vi "GetPower.vi"(4 "error in (no error)":errorcluster, 5 "Measeaurement mode":string(combo)="PM100D", 6 "Wavelength (nm)":dbl=350.0 min=350.0 max=1100.0 format="%#.1f", 7 "Input Device":refnum<visa-resource-name>) -> (0 "error out":errorcluster, 1 "Power (W)":dbl, 2 "Responsivity (A/W)":dbl, 3 "VISA Resource Name out":refnum<visa-resource-name>="GPIB0::22::INSTR")   [LabVIEW 2011]
uses:
  <vilib>/Utility/file.llb/Read From Spreadsheet File (DBL).vi
panel:
  out "Det36A responsivity":dbl[](array[numeric])
  out "Wavelength":dbl[](array[numeric])
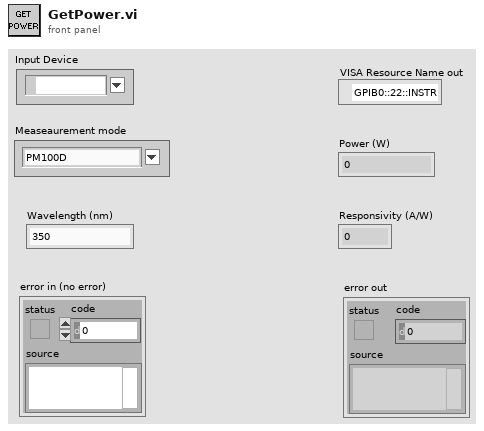
[diagram p1: front panel]
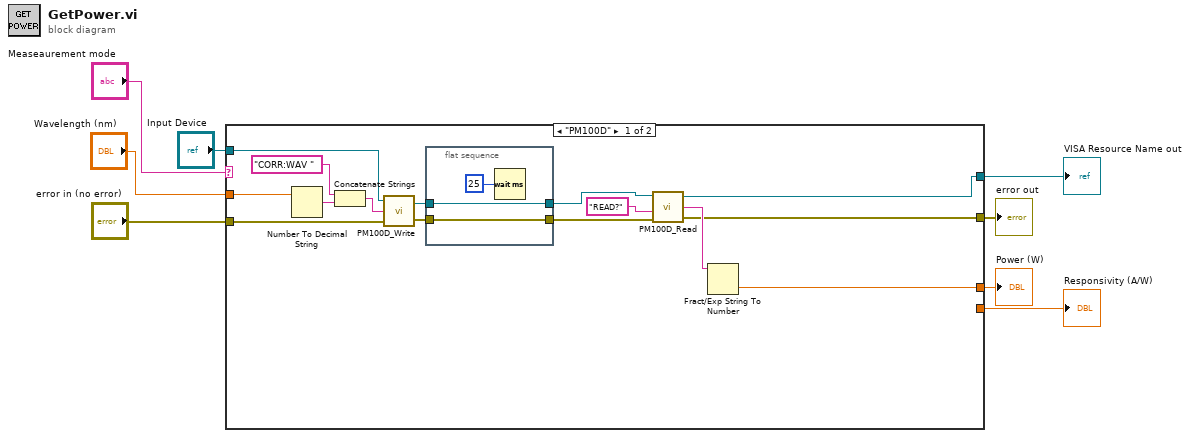
[diagram p0: block diagram]
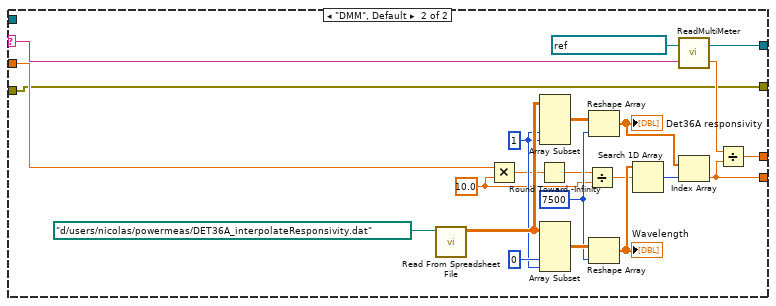
[diagram p2: hidden frame]
diagram:
  n1 = case shown="\"PM100D\"" "Measeaurement mode" {
    selector: "Measeaurement mode" -> [_ w29]
    tunnel: "Input Device" -> [w17 _]
    tunnel: [_ w37] -> w7
    tunnel: [w15 w36] -> w6
    tunnel: "Wavelength (nm)" -> [w19 w35]
    tunnel: [w21 w30] -> w4
    tunnel: [w12 w27] -> w2
    tunnel: "error in (no error)" -> [w9 w27]
    frame "PM100D" {
      n2 = Number To Decimal String(number=w19) -> (decimal integer string=w20:string)  [unwired: 1 in]
      n3 = Concatenate Strings("CORR:WAV " ("chaîne"), w20) -> (w16:string)
      n4 = call "PM100D_Write.vi"("error in (no error)"=w9, "Command"=w16, "VISA in"=w17) -> ("error out"=w10:errorcluster, "VISA out"=w14:refnum<visa-resource-name>)
      n5 = flat-sequence {
        tunnel: w14 -> [w26]
        tunnel: [w26] -> w13
        tunnel: [w24] -> w11
        tunnel: w10 -> [w24]
        frame #0 {
          n6 = Wait (ms)(milliseconds to wait=u32 25) -> ()  [unwired: 1 out]
        }
      }
      n7 = call "PM100D_Read.vi"("error in (no error)"=w11, "Command"="READ?", "VISA in"=w13) -> ("error out"=w12:errorcluster, "ReadValue"=w22:string, "VISA out"=w21:refnum<visa-resource-name>)  [unwired: 1 in]
      n8 = Fract/Exp String To Number(string=w22) -> (number=w15:dbl)  [unwired: 3 in, 1 out]
    }
    frame "DMM", Default {
      w32 = 10.0 ("y")
      w42 = 7500 ("dimension size")
      w44 = 1 ("length")
      n9 = call-poly <vilib>:"Read From Spreadsheet File.vi"("file path (dialog if empty)"=path "d:/users/nicolas/powermeas/DET36A_interpolateResponsivity.dat" ("file (use dialog)")) -> ("all rows"=w45:dbl[][])  [unwired: 6 in, 4 out]
      n10 = Multiply(x=w35, y=w32) -> (x*y=w34:dbl)
      n11 = Round Toward -Infinity(1:w34) -> (0:w33:dbl)
      n12 = Array Subset(array=w45, index (col)=w44, length (col)=w44) -> (w43:dbl[][])  [unwired: 2 in]
      n13 = Array Subset(array=w45, index (col)=0 ("index"), length (col)=w44) -> (w46:dbl[][])  [unwired: 2 in]
      n14 = Divide(x=w33, y=w32) -> (x/y=w31:dbl)
      n15 = Reshape Array(w43, w42) -> (w39:dbl[])
      "Det36A responsivity" <- w39
      n16 = Reshape Array(w46, w42) -> (w41:dbl[])
      "Wavelength" <- w41
      n17 = Search 1D Array(1D array=w41, element=w31) -> (index of element=w40:i32)  [unwired: 1 in]
      n18 = call "ReadMultiMeter.vi"("Measeaurement mode"=w29, "Input Device"=refnum<visa-resource-name> "GPIB0::22::INSTR" ("Gate - K2400")) -> ("Volt"=w38:dbl, "VISA Resource Name out"=w30:refnum<visa-resource-name>)
      n19 = Index Array(array=w39, index=w40) -> (element=w37:dbl)
      n20 = Divide(x=w38, y=w37) -> (x/y=w36:dbl)
    }
  }
  "Responsivity (A/W)" <- w7
  "Power (W)" <- w6
  "VISA Resource Name out" <- w4
  "error out" <- w2
